vi "Get_tracklog_formated_path.vi"(1 "UTC":dbl format="%<%H:%M:%S>t") -> (0 "Formatted path":string)   [LabVIEW 2011]
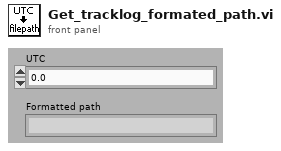
[diagram p1: front panel]
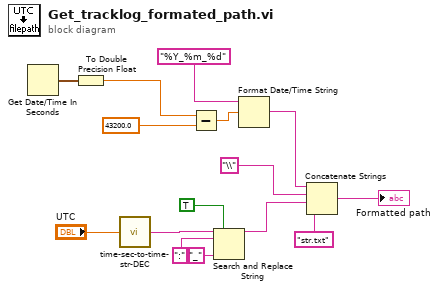
[diagram p0: block diagram]
diagram:
  n1 = Get Date/Time In Seconds() -> (seconds since 1Jan1904=w12:timestamp)
  n2 = To Double Precision Float(number=w12) -> (double precision float=w14:dbl)
  n3 = call "time-sec-to-time-str-DEC.vi"("Numeric"="UTC") -> ("formatted-str"=w6:string)
  n4 = Subtract(x=w14, y=43200.0) -> (x-y=w13:dbl)
  n5 = Search and Replace String(replace all?=TRUE ("replace all? (F)"), input string=w6, search string=":", replace string="_" ("replace string (\"\")")) -> (result string=w4:string)  [unwired: 4 in, 3 out]
  n6 = Format Date/Time String(time format string (%c)="%Y_%m_%d", seconds (now)=w13) -> (date/time string=w10:string)  [unwired: 1 in]
  n7 = Concatenate Strings(w10, "\\" ("string"), w4, "str.txt" ("string")) -> (→"Formatted path":string)
